vi "Initialise Schema.vi"(8 "error in (no error)":errorcluster, 11 "Sqlite Database Manager in":refnum<class "Sqlite Database Manager.lvclass">) -> (0 "error out":errorcluster, 3 "Sqlite Database Manager out":refnum<class "Sqlite Database Manager.lvclass">)   [LabVIEW 2019, in "HierDAL Library.lvlib" / "Database.lvlib" / "Sqlite Database Manager.lvclass"]
uses:
  Sqlite Database Manager.lvclass
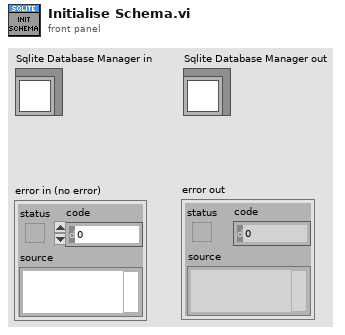
[diagram p1: front panel]
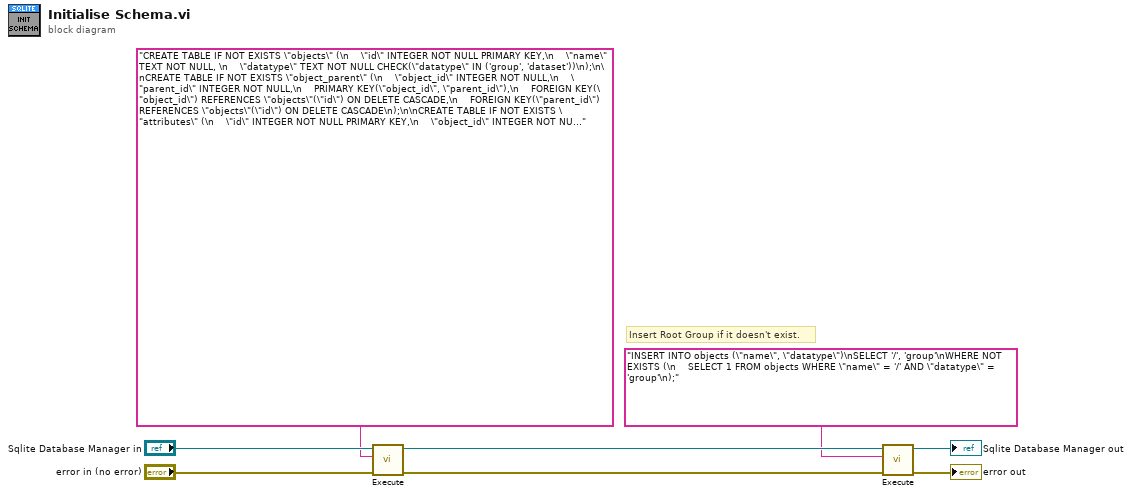
[diagram p0: block diagram]
diagram:
  # "Insert Root Group if it doesn't exist."
  n1 = call-dynamic "Execute.vi"("error in (no error)"="error in (no error)", "Query"="CREATE TABLE IF NOT EXISTS \"objects\" (\n    \"id\" INTEGER NOT NULL PRIMARY KEY,\n    \"name\" TEXT NOT NULL, \n    \"datatype\" TEXT NOT NULL CHECK(\"datatype\" IN ('group', 'dataset'))\n);\n\nCREATE TABLE IF NOT EXISTS \"object_parent\" (\n    \"object_id\" INTEGER NOT NULL,\n    \"parent_id\" INTEGER NOT NULL,\n    PRIMARY KEY(\"object_id\", \"parent_id\"),\n    FOREIGN KEY(\"object_id\") REFERENCES \"objects\"(\"id\") ON DELETE CASCADE,\n    FOREIGN KEY(\"parent_id\") REFERENCES \"objects\"(\"id\") ON DELETE CASCADE\n);\n\nCREATE TABLE IF NOT EXISTS \"attributes\" (\n    \"id\" INTEGER NOT NULL PRIMARY KEY,\n    \"object_id\" INTEGER NOT NULL,\n    \"key\" TEXT NOT NULL,\n    \"value\",\n    UNIQUE(\"object_id\", \"key\"),\n    FOREIGN KEY(\"object_id\") REFERENCES \"objects\"(\"id\") ON DELETE CASCADE\n);\n\nCREATE INDEX IF NOT EXISTS idx_object_parent_object_id ON object_parent(\"object_id\");\nCREATE INDEX IF NOT EXISTS idx_object_parent_parent_id ON object_parent(\"parent_id\");", "Sqlite Database Manager in"="Sqlite Database Manager in") -> ("error out"=w1:errorcluster, "Sqlite Database Manager out"=w6:refnum<class "Sqlite Database Manager.lvclass">)  [unwired: 7 in]
  n2 = call-dynamic "Execute.vi"("error in (no error)"=w1, "Query"="INSERT INTO objects (\"name\", \"datatype\")\nSELECT '/', 'group'\nWHERE NOT EXISTS (\n    SELECT 1 FROM objects WHERE \"name\" = '/' AND \"datatype\" = 'group'\n);", "Sqlite Database Manager in"=w6) -> ("error out"=→"error out":errorcluster, "Sqlite Database Manager out"=→"Sqlite Database Manager out":refnum<class "Sqlite Database Manager.lvclass">)  [unwired: 7 in]
